vi "Actor Core.vi"(8 "error in":errorcluster, 11 "InterferometrUI in":refnum<class "InterferometerUI.lvclass">) -> (0 "error out":errorcluster, 3 "Actor out":refnum<class "Actor.lvclass">)   [LabVIEW 2023, in "InterferometrUI.lvlib" / "InterferometerUI.lvclass"]
doc: "(<B>Filename</B>: Actor Framework.lvlib:Actor.lvclass:Actor Core.vi)\n\nReceives messages to the actor, reacts to them, and initiates any error handling that may shut the actor down.\n\nDescendant classes may override this VI to append parallel tasks for the actor to complete while it handles messages. Overrides use the Call Parent Class Method node."
uses:
  InterferometerUI.lvclass
  InterferometerUI.lvclass/InterferometerUI.ctl
  <vilib>/ActorFramework/Actor/Actor.lvclass
  <vilib>/ActorFramework/Stop Msg/Stop Msg.lvclass
  TranslationStage/ArduinoTranslationStageActor/ArduinoTranslationStage Actor/ArduinoTranslationStage.lvclass
  Cameras_LV/ZWO_ASI/ZWO_ASI/ZWO_ASI.lvclass
  TranslationStage/ArduinoTranslationStageActor/ArduinoTranslationStage Messages/MoveBySteps Msg/MoveBySteps Msg.lvclass
  Cameras_LV/ZWO_ASI/ZWO_ASI Messages/StartCapture Msg/StartCapture Msg.lvclass
  Cameras_LV/ZWO_ASI/ZWO_ASI Messages/StopCapture Msg/StopCapture Msg.lvclass
  Cameras_LV/ZWO_ASI/ZWO_ASI Messages/OpenCamera Msg/OpenCamera Msg.lvclass
  Applications/National Instruments/LabVIEW 2023 64-bit/vi.lib/ActorFramework/Actor/Actor.lvclass
  TranslationStage/ArduinoTranslationStageActor/ArduinoTranslationStage Messages/Init Msg/Init Msg.lvclass
  Users/alexandrosspiliotis/Documents/LV_DAQ_Project/TranslationStage/ArduinoTranslationStageActor/ArduinoTranslationStage Actor/ArduinoTranslationStage.lvclass
  Users/alexandrosspiliotis/Documents/LV_DAQ_Project/Cameras_LV/InitDeinit/InitDeinit.lvclass
  Users/alexandrosspiliotis/Documents/LV_DAQ_Project/TranslationStage/StepperMotorController/StepperMotorController.lvclass
  Users/alexandrosspiliotis/Documents/LV_DAQ_Project/TranslationStage/TranslationStages/TranslationStagesInterface.lvclass
  Users/alexandrosspiliotis/Documents/LV_DAQ_Project/Cameras_LV/ZWO_ASI/ZWO_ASI/ZWO_ASI.lvclass
  Users/alexandrosspiliotis/Documents/LV_DAQ_Project/Cameras_LV/ImagingDevice/ImagingDevice.lvclass
panel:
  in  "FileName":string
  in  "Path":path
  out "VI":refnum<vi>
  out "Image":u16[][](graph)
  in  "Exposure":dbl
  in  "Snap":bool
  in  "Live":bool
  in  "Connect Cam":bool
  in  "Connect Stepper":bool
  in  "VISA resource name":refnum<visa-resource-name>
  in  "Stop Button":bool
  in  "Direction":enum16{"Forward", "Backwards"}(ring)
  in  "Polarity":enum16{"Positive", "Negative"}(ring)
  in  "Move Stepper":bool
  in  "Step Time (us)":u32(slide)=100 min=100 step=10 scale=100.0..10000.0
  in  "Steps":u32(slide)=1 min=1 max=10000 step=1 scale=1.0..10000.0
  in  "Scan Segments":u32(slide) max=100 step=1 scale=0.0..100.0
  in  "Scan":bool
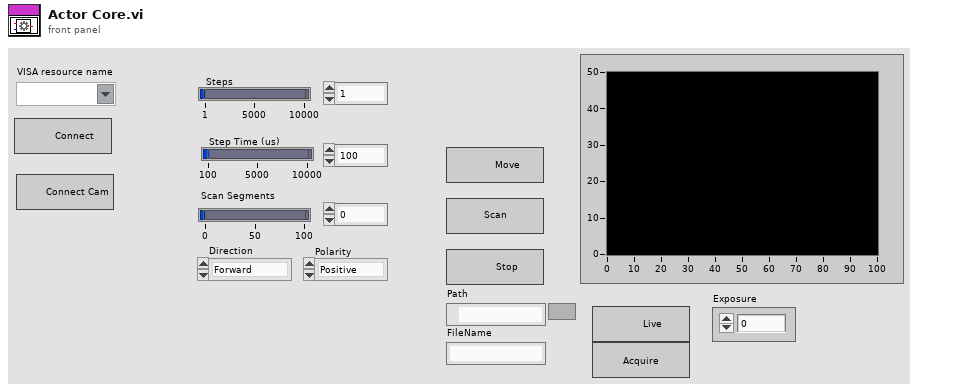
[diagram p1: front panel]
types:
  T1 = enum8{"Enabled", "Disabled", "Disabled and Grayed Out"}
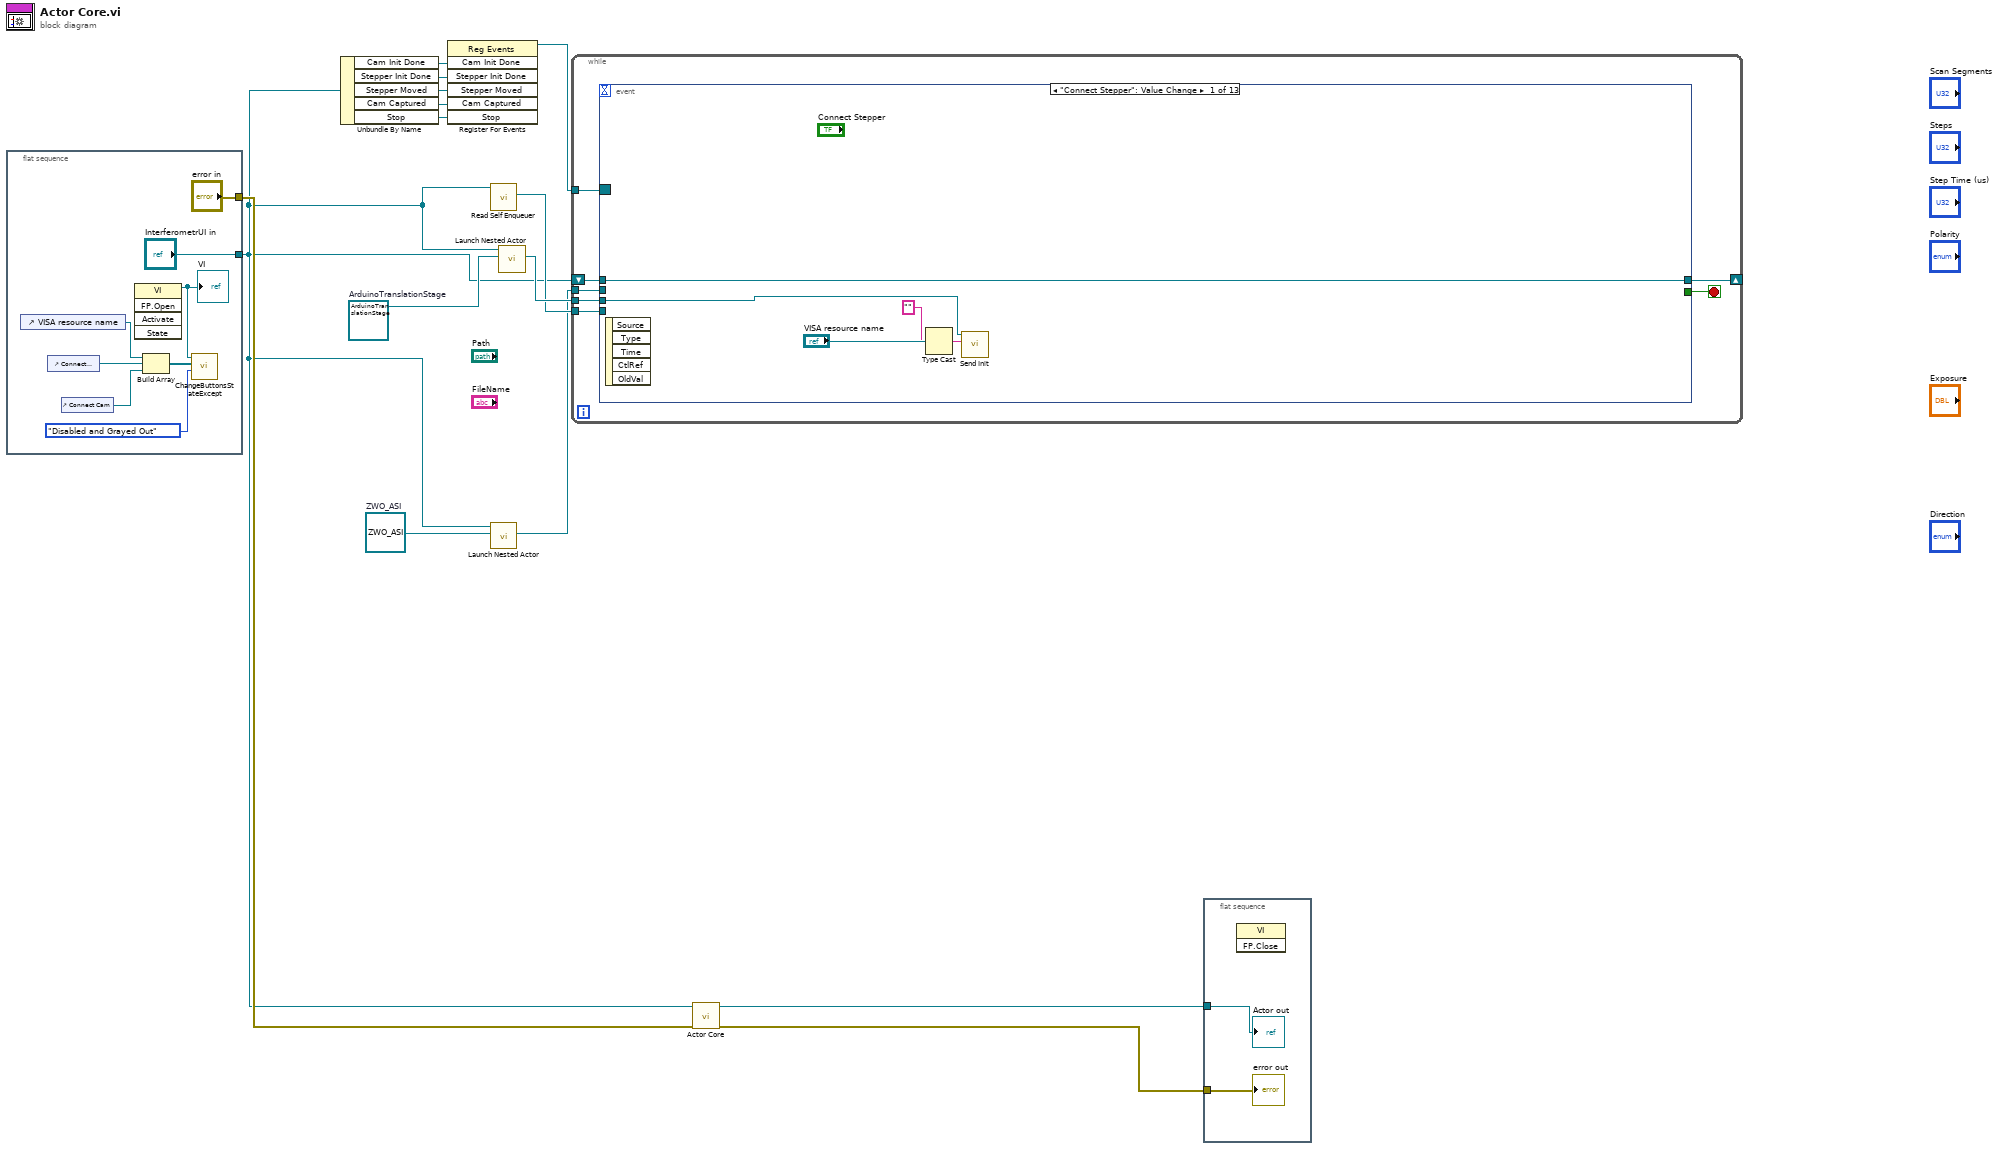
[diagram p0: block diagram]
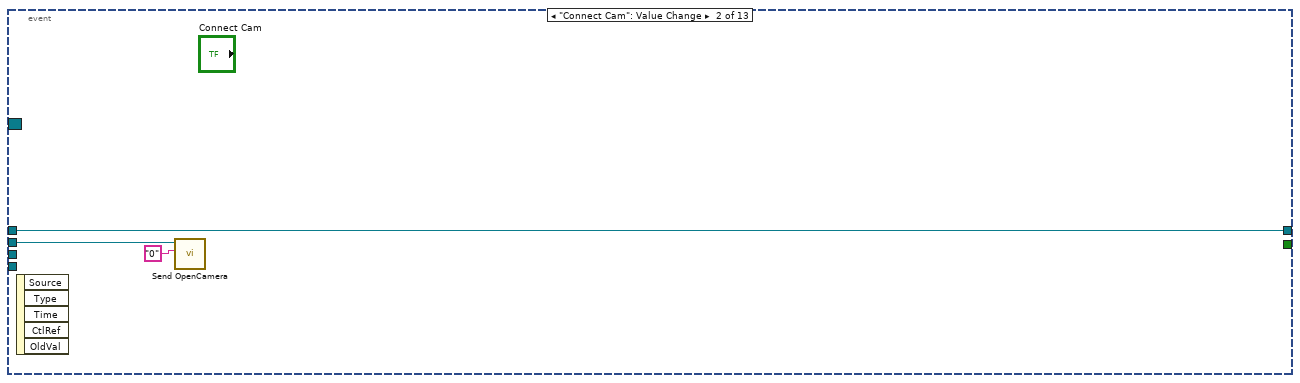
[diagram p2: hidden frame]
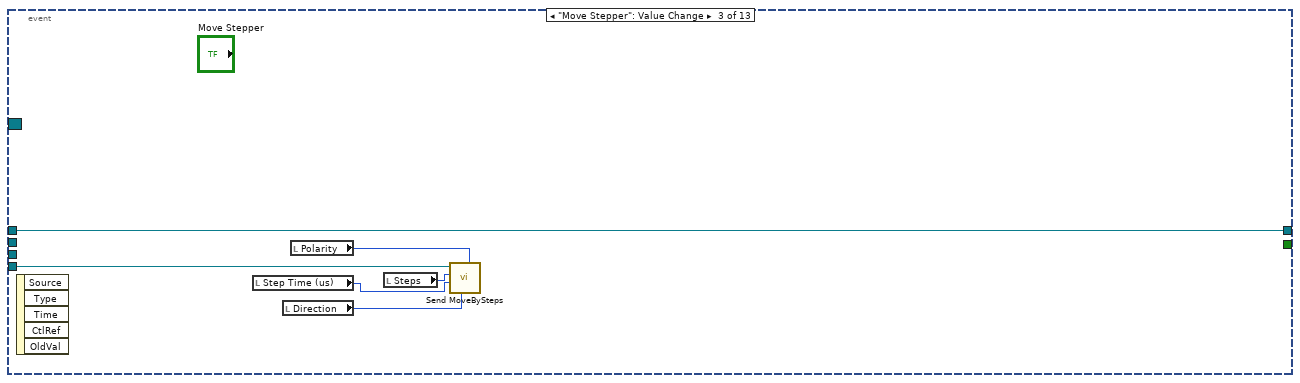
[diagram p3: hidden frame]
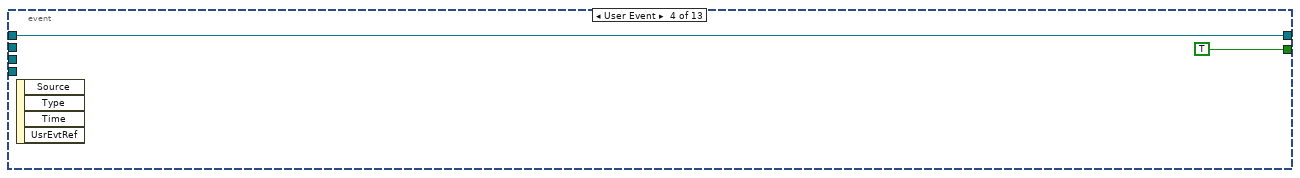
[diagram p4: hidden frame]
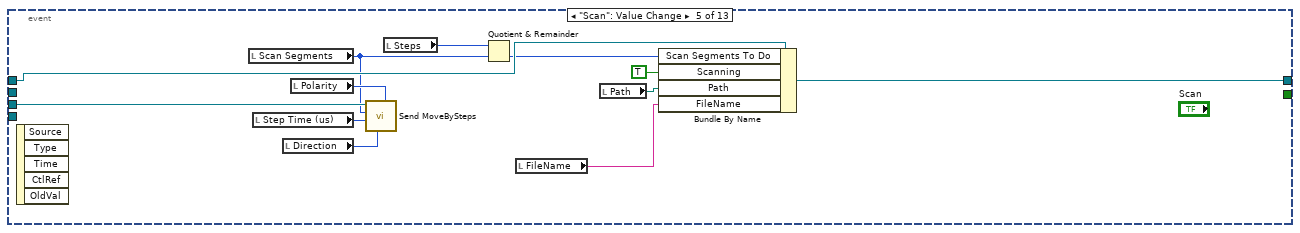
[diagram p5: hidden frame]
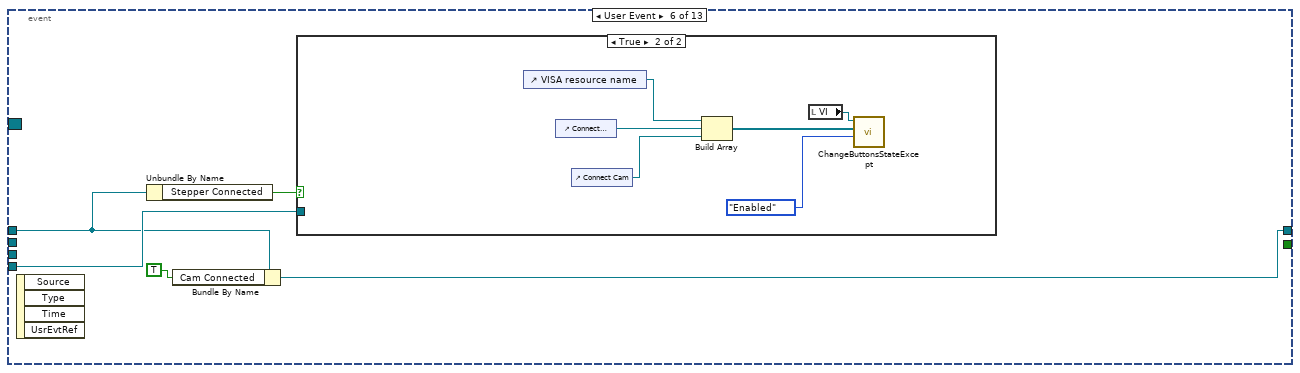
[diagram p6: hidden frame]
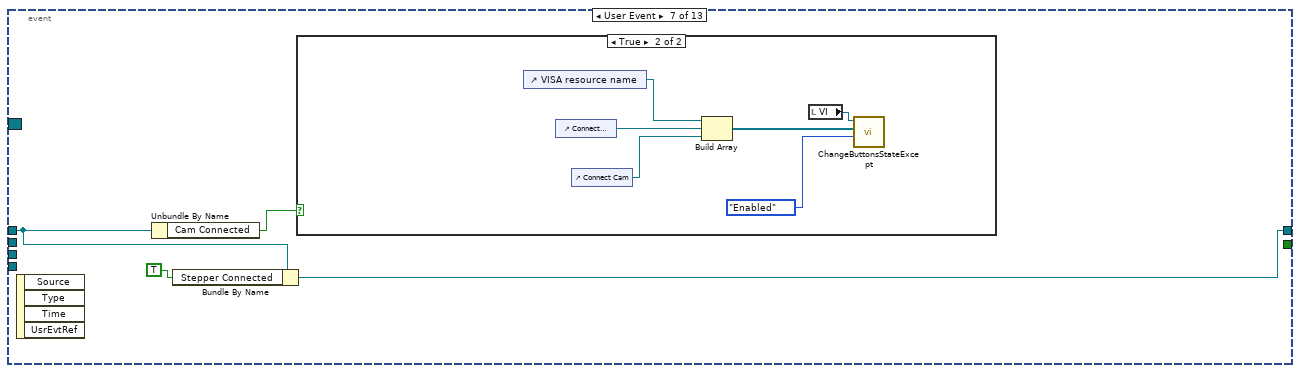
[diagram p8: hidden frame]
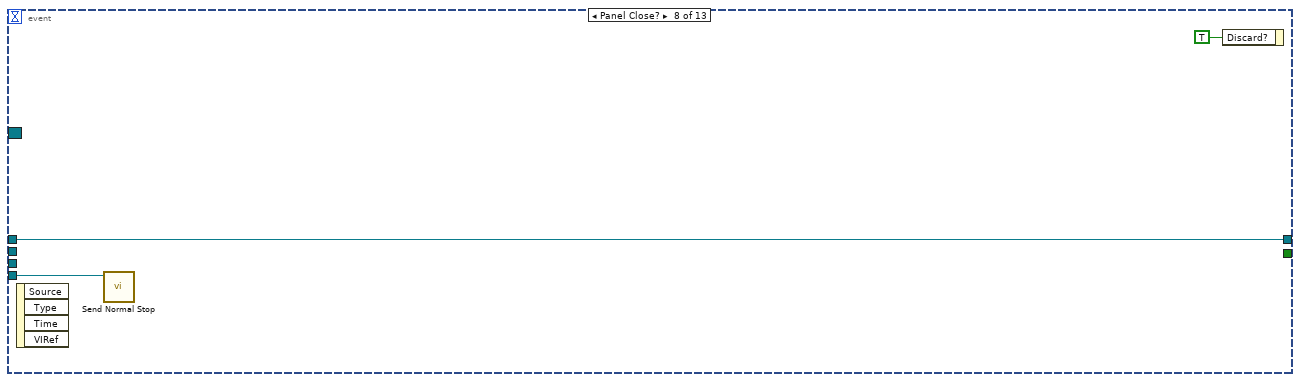
[diagram p10: hidden frame]
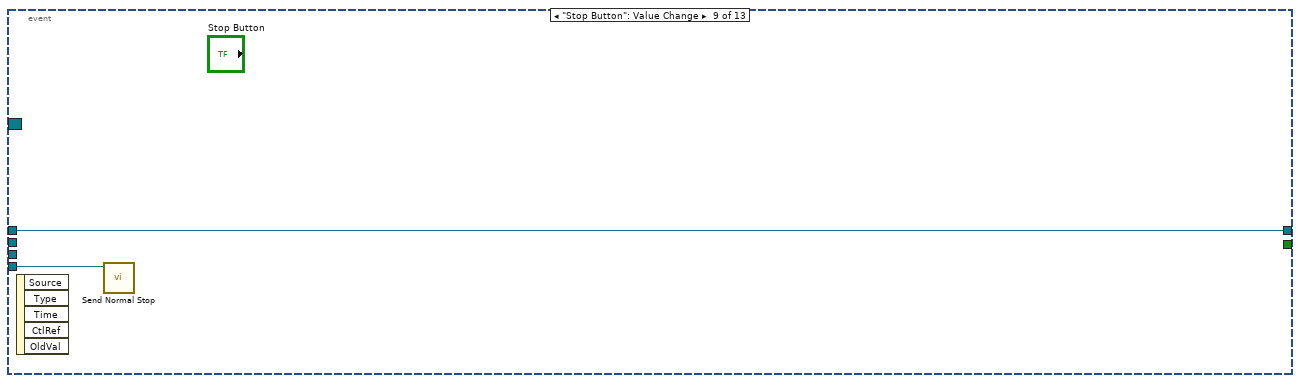
[diagram p11: hidden frame]
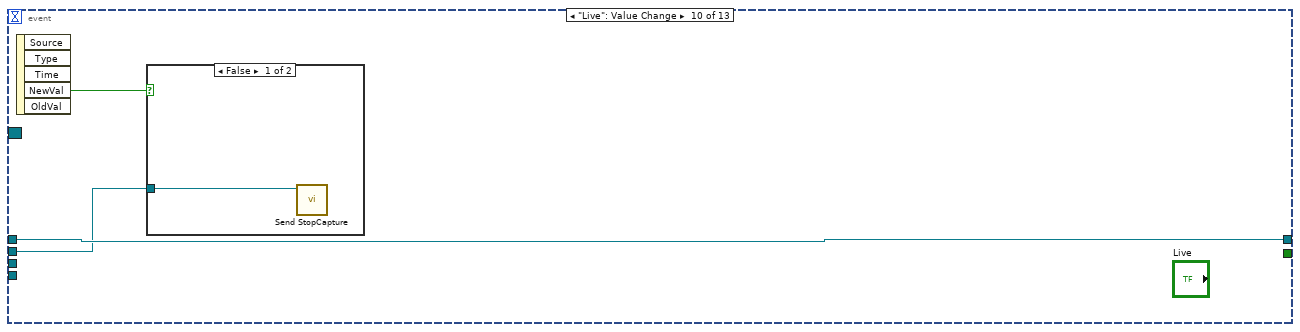
[diagram p12: hidden frame]
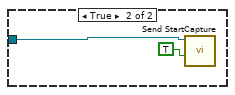
[diagram p13: hidden frame]
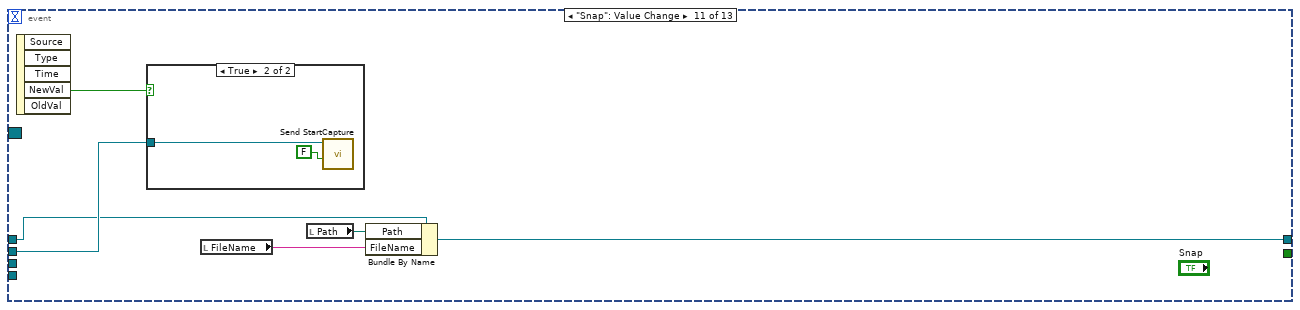
[diagram p14: hidden frame]
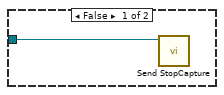
[diagram p15: hidden frame]
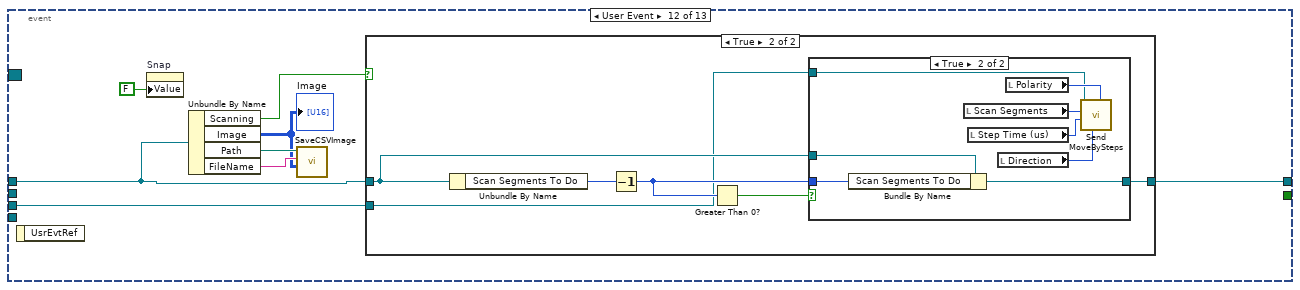
[diagram p16: hidden frame]
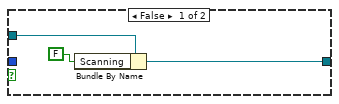
[diagram p18: hidden frame]
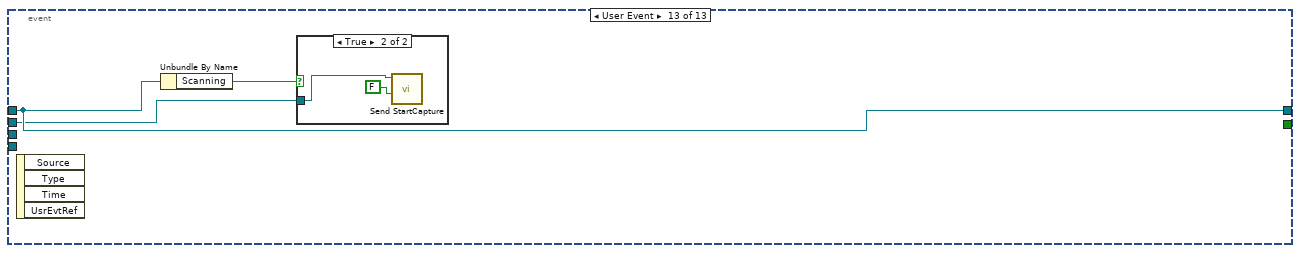
[diagram p19: hidden frame]
diagram:
  w8 = refnum<class "ZWO_ASI.lvclass"> refnum  # ZWO_ASI
  w9 = refnum<class "ArduinoTranslationStage.lvclass"> refnum  # ArduinoTranslationStage
  n1 = flat-sequence {
    tunnel: ["error in"] -> w13
    tunnel: ["InterferometrUI in"] -> w6
    frame #0 {
      n2 = control-ref of="VISA resource name"() -> (w19:refnum<vi>)
      n3 = control-ref of="Connect Stepper"() -> (w20:refnum<vi>)
      n4 = control-ref of="Connect Cam"() -> (w21:refnum<vi>)
      n5 = invoke class="VI" method="FP.Open"() -> (reference out=w16:refnum<vi>)  [unwired: 5 in, 4 out]
      "VI" <- w16
      n6 = Build Array(w19, w20, w21) -> (w18:refnum<vi>[])
      n7 = call "ChangeButtonsStateExcept.vi"("Disabled"=T1."Disabled and Grayed Out", "Exceptions"=w18, "VI in"=w16) -> ()  [unwired: 9 in]
    }
  }
  n8 = Unbundle By Name(w6) -> ("Cam Init Done"=w4:refnum<user-event>, "Stepper Init Done"=w5:refnum<user-event>, "Stepper Moved"=w3:refnum<user-event>, "Cam Captured"=w2:refnum<user-event>, "Stop"=w1:refnum<user-event>)
  n9 = register-events(w4, w5, w3, w2, w1) -> (reference out=w7:refnum<event-registration>)  [unwired: 2 in, 1 out]
  n10 = call <vilib>:"Read Self Enqueuer.vi"("Actor"=w6) -> ("Self Enqueuer"=w11:refnum<class "Message Enqueuer.lvclass">)  [unwired: 10 in]
  n11 = call <vilib>:"Launch Nested Actor.vi"("Nested Actor"=w8, "Caller Actor in"=w6) -> ("Nested Actor's Enqueuer"=w10:refnum<class "Message Enqueuer.lvclass">)  [unwired: 7 in, 2 out]
  n12 = call <vilib>:"Launch Nested Actor.vi"("Nested Actor"=w9, "Caller Actor in"=w6) -> ("Nested Actor's Enqueuer"=w12:refnum<class "Message Enqueuer.lvclass">)  [unwired: 7 in, 2 out]
  n13 = while {
    tunnel: w12 -> [w27]
    tunnel: w11 -> [w28]
    tunnel: w10 -> [w24]
    shift-right: [w30] -> _
    shift-left: w6 -> [w29]
    tunnel: w7 -> [w26]
    stop <- w25 stop-if-true
    n14 = event shown="[0] \"Connect Stepper\": Value Change" {
      selector: w26 -> [_ _ _ _ _ _ _ _ _ _ _ _ _]
      dyn-events: _ -> [_ _ _ _ _ _ _ _ _ _ _ _ _]
      timeout: _ -> [_ _ _ _ _ _ _ _ _ _ _ _ _]
      tunnel: [w35 w38 w44 w46 w57 w62 w72 w82 w84 w87 w91 w104 w128] -> w30
      tunnel: w29 -> [w35 w38 w44 w46 w56 w59 w71 w82 w84 w87 w94 w105 w128]
      tunnel: w28 -> [_ _ w39 _ _ w60 _ w81 w83 _ _ _ _]
      tunnel: w27 -> [w32 _ _ _ w52 _ _ _ _ _ _ w100 _]
      tunnel: [_ _ _ TRUE _ _ _ _ _ _ _ _ _] -> w25
      tunnel: w24 -> [_ w37 _ _ _ _ _ _ _ w86 w96 _ w126]
      event "Connect Stepper": Value Change {
        n15 = event-data() -> ()  [unwired: 1 in, 5 out]
        n16 = Type Cast(type="", x="VISA resource name") -> (*(type *) &x=w31:string)
        n17 = call "Send Init.vi"("Address"=w31, "Message Enqueuer"=w32) -> ()  [unwired: 8 in, 2 out]
      }
      event "Connect Cam": Value Change {
        n18 = event-data() -> ()  [unwired: 1 in, 5 out]
        n19 = call "Send OpenCamera.vi"("Camera ID"="0", "Message Enqueuer"=w37) -> ()  [unwired: 8 in, 2 out]
      }
      event "Move Stepper": Value Change {
        n20 = event-data() -> ()  [unwired: 1 in, 5 out]
        n21 = local read "Step Time (us)"() -> (w42:u32)
        n22 = local read "Direction"() -> (w40:enum16{"Forward", "Backwards"})
        n23 = local read "Polarity"() -> (w41:enum16{"Positive", "Negative"})
        n24 = local read "Steps"() -> (w43:u32)
        n25 = call "Send MoveBySteps.vi"("Polarity"=w41, "Direction"=w40, "Speed"=w42, "Steps"=w43, "Message Enqueuer"=w39) -> ()  [unwired: 5 in, 2 out]
      }
      event User Event {
        n26 = event-data() -> ()  [unwired: 1 in, 4 out]
      }
      event "Scan": Value Change {
        n27 = event-data() -> ()  [unwired: 1 in, 5 out]
        n28 = local read "Scan Segments"() -> (w50:u32)
        n29 = local read "Step Time (us)"() -> (w55:u32)
        n30 = local read "Direction"() -> (w53:enum16{"Forward", "Backwards"})
        n31 = local read "Polarity"() -> (w54:enum16{"Positive", "Negative"})
        n32 = call "Send MoveBySteps.vi"("Polarity"=w54, "Direction"=w53, "Speed"=w55, "Steps"=w50, "Message Enqueuer"=w52) -> ()  [unwired: 5 in, 2 out]
        n33 = local read "Steps"() -> (w51:u32)
        n34 = Quotient & Remainder(x=w51, y=w50) -> (floor(x/y)=w49:u32)  [unwired: 1 out]
        n35 = local read "FileName"() -> (w47:string)
        n36 = local read "Path"() -> (w48:path)
        n37 = Bundle By Name(cluster=w56, "Scan Segments To Do"=w49, "Scanning"=TRUE, "Path"=w48, "FileName"=w47) -> (w57:refnum<class "InterferometerUI.lvclass">)
      }
      event User Event {
        n38 = event-data() -> ()  [unwired: 1 in, 4 out]
        n39 = Unbundle By Name(w59) -> ("Stepper Connected"=w61:bool)
        n40 = Bundle By Name(cluster=w59, "Cam Connected"=TRUE) -> (w62:refnum<class "InterferometerUI.lvclass">)
        n41 = case shown="True" w61 {
          tunnel: w60 -> [_ _]
          frame False {
          }
          frame True {
            n42 = control-ref of="VISA resource name"() -> (w68:refnum<vi>)
            n43 = control-ref of="Connect Stepper"() -> (w67:refnum<vi>)
            n44 = control-ref of="Connect Cam"() -> (w66:refnum<vi>)
            n45 = Build Array(w68, w67, w66) -> (w69:refnum<vi>[])
            n46 = local read "VI"() -> (w65:refnum<vi>)
            n47 = call "ChangeButtonsStateExcept.vi"("Disabled"=T1."Enabled", "Exceptions"=w69, "VI in"=w65) -> ()  [unwired: 9 in]
          }
        }
      }
      event User Event {
        n48 = event-data() -> ()  [unwired: 1 in, 4 out]
        n49 = Unbundle By Name(w71) -> ("Cam Connected"=w70:bool)
        n50 = Bundle By Name(cluster=w71, "Stepper Connected"=TRUE ("Cam Connected")) -> (w72:refnum<class "InterferometerUI.lvclass">)
        n51 = case shown="True" w70 {
          frame False {
          }
          frame True {
            n52 = control-ref of="VISA resource name"() -> (w78:refnum<vi>)
            n53 = control-ref of="Connect Stepper"() -> (w77:refnum<vi>)
            n54 = control-ref of="Connect Cam"() -> (w76:refnum<vi>)
            n55 = Build Array(w78, w77, w76) -> (w79:refnum<vi>[])
            n56 = local read "VI"() -> (w75:refnum<vi>)
            n57 = call "ChangeButtonsStateExcept.vi"("Disabled"=T1."Enabled", "Exceptions"=w79, "VI in"=w75) -> ()  [unwired: 9 in]
          }
        }
      }
      event Panel Close? {
        n58 = event-data() -> ()  [unwired: 1 in, 4 out]
        n59 = call <vilib>:"Send Normal Stop.vi"("Message Enqueuer"=w81) -> ()  [unwired: 10 in, 1 out]
        n60 = event-data("Discard?"=TRUE) -> ()  [unwired: 1 in, 1 out]
      }
      event "Stop Button": Value Change {
        n61 = event-data() -> ()  [unwired: 1 in, 5 out]
        n62 = call <vilib>:"Send Normal Stop.vi"("Message Enqueuer"=w83) -> ()  [unwired: 10 in, 1 out]
      }
      event "Live": Value Change {
        n63 = event-data() -> ("NewVal"=w85:bool)  [unwired: 1 in, 4 out]
        n64 = case shown="False" w85 {
          tunnel: w86 -> [w88 w90]
          frame False {
            n65 = call "Send StopCapture.vi"("Message Enqueuer"=w88) -> ()  [unwired: 9 in, 2 out]
          }
          frame True {
            n66 = call "Send StartCapture.vi"("Continuous"=TRUE, "Message Enqueuer"=w90) -> ()  [unwired: 8 in, 2 out]
          }
        }
      }
      event "Snap": Value Change {
        n67 = event-data() -> ("NewVal"=w95:bool)  [unwired: 1 in, 4 out]
        n68 = case shown="True" w95 {
          tunnel: w96 -> [w97 w99]
          frame False {
            n69 = call "Send StopCapture.vi"("Message Enqueuer"=w97) -> ()  [unwired: 9 in, 2 out]
          }
          frame True {
            n70 = call "Send StartCapture.vi"("Continuous"=FALSE, "Message Enqueuer"=w99) -> ()  [unwired: 8 in, 2 out]
          }
        }
        n71 = local read "FileName"() -> (w92:string)
        n72 = local read "Path"() -> (w93:path)
        n73 = Bundle By Name(cluster=w94, "Path"=w93, "FileName"=w92) -> (w91:refnum<class "InterferometerUI.lvclass">)
      }
      event User Event {
        n74 = event-data() -> ()  [unwired: 1 in, 1 out]
        n75 = property on="Snap" class="Bool (strict)"("Value"=FALSE ("Snap")) -> ()  [unwired: 2 in, 2 out]
        n76 = Unbundle By Name(w105) -> ("Scanning"=w106:bool, "Image"=w101:u16[][], "Path"=w103:path, "FileName"=w102:string)
        "Image" <- w101
        n77 = call "SaveCSVImage.vi"("Image"=w101, "FileName"=w102, "Path"=w103) -> ()  [unwired: 9 in]
        n78 = case shown="True" w106 {
          tunnel: w105 -> [w108 w113]
          tunnel: [w108 w114] -> w104
          tunnel: w100 -> [_ w109]
          frame False {
          }
          frame True {
            n79 = Unbundle By Name(w113) -> ("Scan Segments To Do"=w112:u16)
            n80 = Decrement(x=w112) -> (x-1=w111:u16)
            n81 = Greater Than 0?(x=w111) -> (x > 0?=w110:bool)
            n82 = case shown="True" w110 {
              tunnel: [w115 w122] -> w114
              tunnel: w113 -> [w117 w120]
              tunnel: w111 -> [_ w119]
              tunnel: w109 -> [_ w118]
              frame False {
                n83 = Bundle By Name(cluster=w117, "Scanning"=FALSE) -> (w115:refnum<class "InterferometerUI.lvclass">)
              }
              frame True {
                n84 = Bundle By Name(cluster=w120, "Scan Segments To Do"=w119) -> (w122:refnum<class "InterferometerUI.lvclass">)
                n85 = local read "Scan Segments"() -> (w121:u32)
                n86 = local read "Step Time (us)"() -> (w125:u32)
                n87 = local read "Direction"() -> (w123:enum16{"Forward", "Backwards"})
                n88 = local read "Polarity"() -> (w124:enum16{"Positive", "Negative"})
                n89 = call "Send MoveBySteps.vi"("Polarity"=w124, "Direction"=w123, "Speed"=w125, "Steps"=w121, "Message Enqueuer"=w118) -> ()  [unwired: 5 in, 2 out]
              }
            }
          }
        }
      }
      event User Event {
        n90 = event-data() -> ()  [unwired: 1 in, 4 out]
        n91 = Unbundle By Name(w128) -> ("Scanning"=w127:bool)
        n92 = case shown="True" w127 {
          tunnel: w126 -> [_ w130]
          frame False {
          }
          frame True {
            n93 = call "Send StartCapture.vi"("Continuous"=FALSE, "Message Enqueuer"=w130) -> ()  [unwired: 8 in, 2 out]
          }
        }
      }
    }
  }
  n94 = call-parent "Actor Core.vi"("error in"=w13, "Actor in"=w6) -> ("error out"=w15:errorcluster, "Actor out"=w14:refnum<class "Actor.lvclass">)  [unwired: 8 in]
  n95 = flat-sequence {
    tunnel: w15 -> [w132]
    tunnel: w14 -> [w131]
    frame #0 {
      n96 = invoke class="VI" method="FP.Close"() -> ()  [unwired: 3 in, 3 out]
      "error out" <- w132
      "Actor out" <- w131
    }
  }
